vi "Display.vi"(8 "error in":errorcluster, 11 "Timeout One Button in":refnum<class "Timeout One Button.lvclass">) -> (0 "error out":errorcluster, 3 "Timeout One Button out":refnum<class "Timeout One Button.lvclass">)   [LabVIEW 2021, in "Pop-Up.lvlib" / "Timeout One Button.lvclass"]
doc: "This vi displays the one button timeout popup.\n\n<b>Code Developed By:</b> +\nDaniel Coons +\nhttps://github.com/danielcoons/tsc-pop-up"
uses:
  Timeout One Button.lvclass
  C:/Development/Open Source/tsc-pop-up/Popup/Popup.lvclass
  Timeout One Button.lvclass/Timeout One Button.ctl
  Popup/Popup.lvclass/Popup.ctl
  Popup/Data Member Access/Read Theme.vi
  Theme/Theme.lvclass
  Popup/Popup.lvclass
  user32.dll
panel:
  in  "OK Button":bool
  out "header":bool
  out "String":string
  out "count":string
  out "2D Picture":picture
  # "This VI displays the popup"
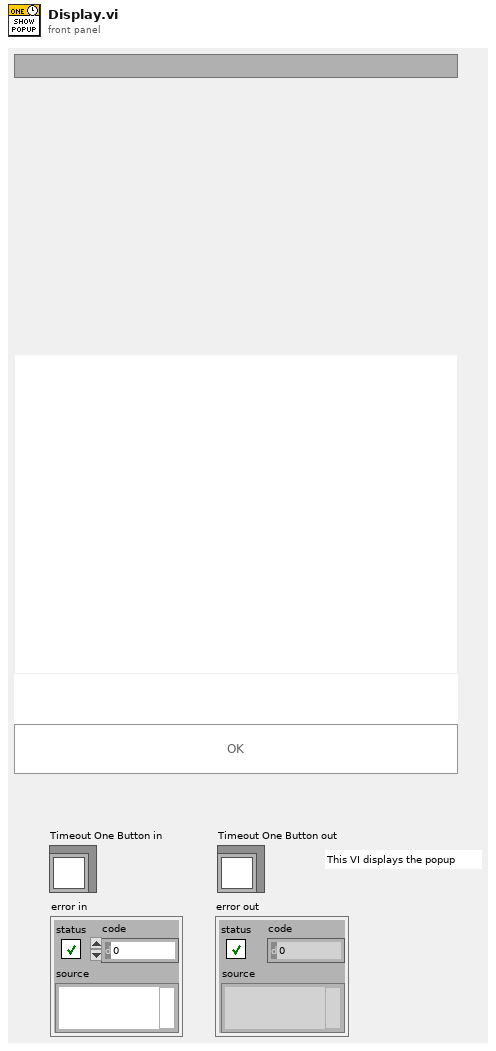
[diagram p1: front panel]
types:
  T1 = typedef "LVPoint32TypeDef.ctl" = cluster{"Horizontal":i32, "Vertical":i32}
  T2 = typedef "LVPositionTypeDef.ctl" = cluster{"Left":i32, "Top":i32}
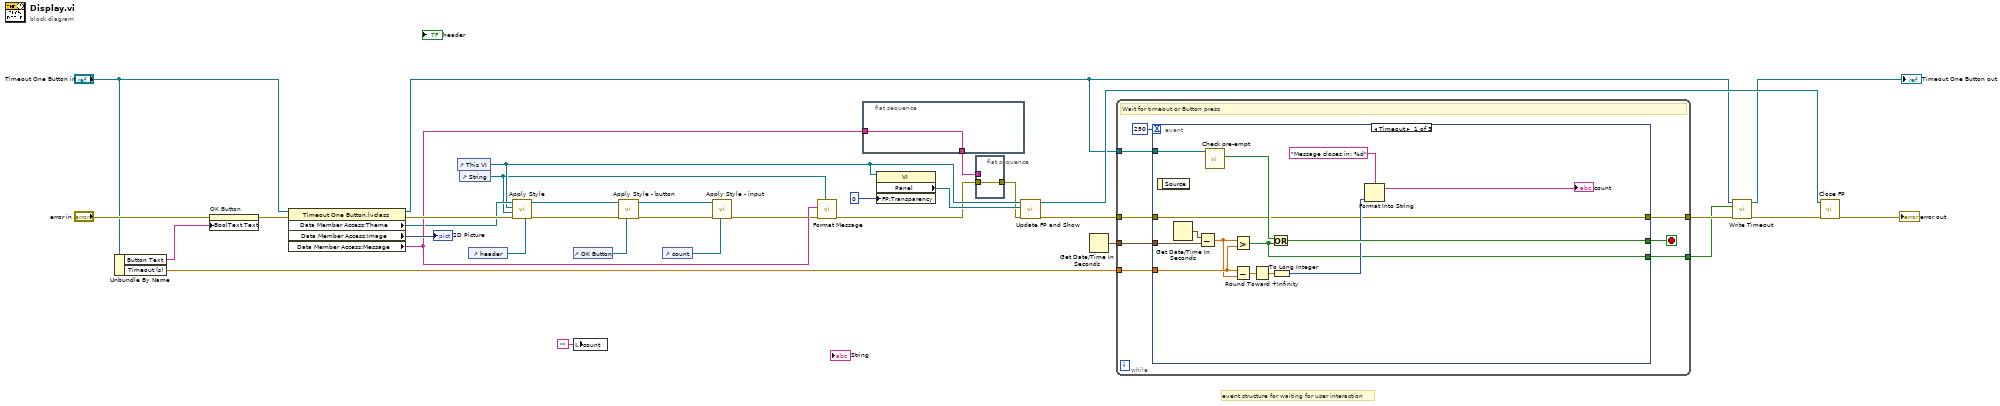
[diagram p0: block diagram]
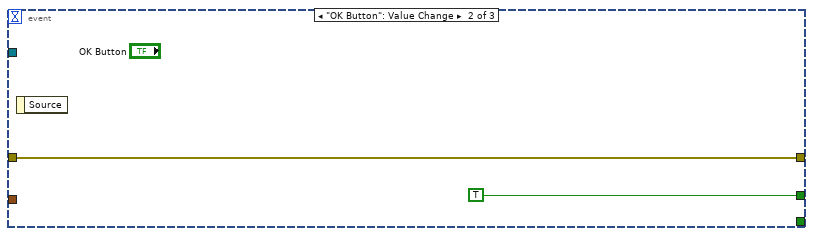
[diagram p2: hidden frame]
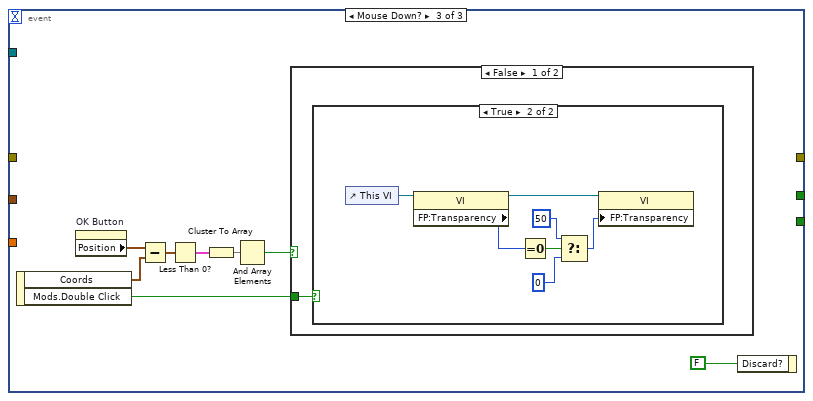
[diagram p3: hidden frame]
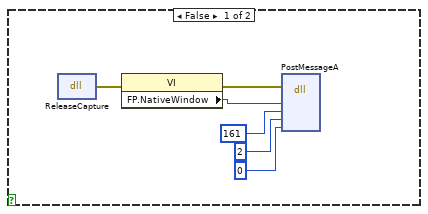
[diagram p4: hidden frame]
diagram:
  # "event structure for waiting for user interaction"
  n1 = Unbundle By Name("Timeout One Button in") -> ("Button Text"=w30:string, "Timeout (s)"=w31:dbl)
  n2 = property on="OK Button" class="Bool"(error in="error in", "BoolText.Text"=w30) -> (error out=w28:errorcluster)  [unwired: 1 in, 1 out]
  n3 = property on="Property Node" class="Timeout One Button.lvclass"(reference="Timeout One Button in", error in=w28) -> (reference out=w1:refnum<class "Timeout One Button.lvclass">, error out=w29:errorcluster, "Data Member Access:Theme"=w20:refnum<class "Theme.lvclass">, "Data Member Access:Image"=→"2D Picture":picture, "Data Member Access:Message"=w22:string)
  n4 = control-ref of="This VI"() -> (w19:refnum<vi>)
  n5 = control-ref of="String"() -> (w18:refnum<vi>)
  n6 = control-ref of="header"() -> (w17:refnum<vi>)
  n7 = call "Apply Style.vi"("header ref"=w17, "error in"=w29, "message ref"=w18, "pop up ref"=w19, "Theme in"=w20) -> ("error out"=w21:errorcluster, "Theme out"=w15:refnum<class "Theme.lvclass">)  [unwired: 5 in]
  n8 = local write "count"("" ("count")) -> ()
  n9 = control-ref of="OK Button"() -> (w14:refnum<vi>)
  n10 = call "Apply Style - button.vi"("button ref"=w14, "error in"=w21, "Theme in"=w15) -> ("error out"=w16:errorcluster, "Theme out"=w12:refnum<class "Theme.lvclass">)  [unwired: 7 in]
  n11 = control-ref of="count"() -> (w11:refnum<vi>)
  n12 = call "Apply Style - input.vi"("input ref"=w11, "error in (no error)"=w16, "Theme in"=w12) -> ("error out"=w13:errorcluster)  [unwired: 7 in, 1 out]
  n13 = call "Format Message.vi"("formatted string"=w18, "error in"=w13, "String Input"=w22) -> ("error out"=w3:errorcluster)  [unwired: 7 in, 1 out]
  n14 = flat-sequence {
    tunnel: [w35] -> w2
    tunnel: w22 -> [w35]
    frame #0 {
    }
  }
  n15 = property on="Property Node" class="VI"(reference=w19, "FP:Transparency"=u8 0 ("Front Panel Window:Transparency")) -> ("Panel"=w25:refnum<vi>)  [unwired: 1 in, 2 out]
  n16 = flat-sequence {
    tunnel: w3 -> [w36]
    tunnel: [w36] -> w4
    tunnel: w2 -> [_]
    frame #0 {
    }
  }
  n17 = call "Update FP and Show.vi"("error in (no error)"=w4, "Panel Ref"=w25, "VI in"=w19) -> ("error out"=w10:errorcluster, "VI out"=w23:refnum<vi>)  [unwired: 7 in]
  n18 = Get Date/Time In Seconds() -> (seconds since 1Jan1904=w32:timestamp)
  n19 = while {
    tunnel: w10 -> [w40]
    tunnel: [w39] -> w33
    tunnel: w32 -> [w44]
    tunnel: w31 -> [w42]
    tunnel: w1 -> [w38]
    tunnel: [w37] -> w5
    stop <- w43 stop-if-true
    # "Wait for timeout or Button press"
    n20 = event shown="[0] Timeout" {
      selector: _ -> [_ _ _]
      dyn-events: _ -> [_ _ _]
      timeout: 250 -> [_ _ _]
      tunnel: w44 -> [w57 _ _]
      tunnel: [w52 TRUE _] -> w43
      tunnel: w42 -> [w56 _ _]
      tunnel: w40 -> [w48 w60 _]
      tunnel: [w48 w60 _] -> w39
      tunnel: w38 -> [w50 _ _]
      tunnel: [w45 _ _] -> w37
      event Timeout {
        n21 = event-data() -> ()  [unwired: 1 in, 1 out]
        n22 = Get Date/Time In Seconds() -> (seconds since 1Jan1904=w58:timestamp)
        n23 = Subtract(x=w58, y=w57) -> (x-y=w55:dbl)
        n24 = call "Check pre-empt.vi"("_Popup in"=w50) -> ("Pre-empted?"=w51:bool)  [unwired: 8 in, 2 out]
        n25 = Greater?(x=w55, y=w56) -> (0:w45:bool)
        n26 = Subtract(x=w56, y=w55) -> (x-y=w54:dbl)
        n27 = Round Toward +Infinity(x=w54) -> (ceil(x): smallest int >= x=w47:dbl)
        n28 = Or(x=w51, y=w45) -> (x .or. y?=w52:bool)
        n29 = To Long Integer(number=w47) -> (32bit integer=w49:i32)
        n30 = Format Into String(format string="Message closes in: %d", w49) -> (resulting string=→"count":string)  [unwired: 2 in, 1 out]
      }
      event "OK Button": Value Change {
        n31 = event-data() -> ()  [unwired: 1 in, 1 out]
      }
      event Mouse Down? {
        n32 = event-data() -> ("Coords"=w63:T1, "Mods.Double Click"=w61:bool)  [unwired: 1 in]
        n33 = property on="OK Button" class="Bool"() -> ("Position"=w67:T2)  [unwired: 2 in, 2 out]
        n34 = Subtract(x=w67, y=w63) -> (x-y=w66:T2)
        n35 = Less Than 0?(x=w66) -> (x < 0?=w65:cluster{"Left":bool, "Top":bool})
        n36 = Cluster To Array(cluster=w65) -> (array=w64:bool[])
        n37 = And Array Elements(Boolean array=w64) -> (logical AND=w62:bool)
        n38 = case shown="False" w62 {
          tunnel: w61 -> [w69 _]
          frame False {
            n39 = case shown="True" w69 {
              frame False {
                n40 = dll-call lib="user32.dll" fn="ReleaseCapture"() -> (error out=w73:errorcluster)  [unwired: 4 in, 1 out]
                n41 = property on="Property Node" class="VI"(error in=w73) -> (error out=w74:errorcluster, "FP.NativeWindow"=w75:u64)  [unwired: 1 in, 1 out]
                n42 = dll-call lib="user32.dll" fn="PostMessageA"(error in=w74, "hWnd"=w75, "Msg"=161, "wParam"=2, "lParam"=0) -> ()  [unwired: 7 in, 2 out]
              }
              frame True {
                n43 = control-ref of="This VI"() -> (w82:refnum<vi>)
                n44 = property on="Property Node" class="VI"(reference=w82) -> (reference out=w80:refnum<vi>, "FP:Transparency"=w81:u8)  [unwired: 1 in, 1 out]
                n45 = Equal To 0?(x=w81) -> (x = 0?=w79:bool)
                n46 = Select(t=u8 50, s=w79, f=u8 0) -> (s? t:f=w78:u8)
                n47 = property on="Property Node" class="VI"(reference=w80, "FP:Transparency"=w78) -> ()  [unwired: 1 in, 2 out]
              }
            }
          }
          frame True {
          }
        }
        n48 = event-data ("Event Filter Node")("Discard?"=FALSE) -> ()  [unwired: 1 in, 1 out]
      }
    }
  }
  n49 = call "Write Timeout.vi"("error in"=w33, "Timeout?"=w5, "Popup in"=w1) -> ("error out"=w7:errorcluster, "Popup out"=→"Timeout One Button out":refnum<class "Timeout One Button.lvclass">)  [unwired: 7 in]
  n50 = call "Close FP.vi"("error in (no error)"=w7, "VI in"=w23) -> ("error out"=→"error out":errorcluster)  [unwired: 9 in]
